vi "Merge Image Data with mask.vi"(6 "Col":i32=1, 7 "Row":i32=1, 9 "Mask":u8[][](array[numeric])=[[0, 1, 1], [1, 0, 1], [1, 1, 1]], 10 "Image Data 2":u16[][](array[numeric])=[[2, 2, 2], [2, 2, 2], [2, 2, 2]] format="%.0x", 11 "Image Data 1":u16[][](array[numeric])=[[0, 0, 0, 0, 0, 0, 0, 0, 0, 0, 0, 0, 0, 0, 0, 0], [0, 3, 3, 3, 0, 0, 0, 0, 0, 0, 0, 0, 0, 0, 0, 0], [0, 3, 3, 3, 0, 0, 0, 0, 0, 0, 0, 0, 0, 0, 0, 0], [0, 3, 3, 3, 0, 0, 0, 0, 0, 0, 0, 0, 0, 0, 0, 0], [0, 0, 0, 0, 0, 0, 0, 0, 0, 0, 0, 0, 0, 0, 0, 0], [0, 0, 0, 0, 0, 0, 0, 0, 0, 0, 0, 0, 0, 0, 0, 0], [0, 0, 0, 0, 0, 0, 0, 0, 0, 0, 0, 0, 0, 0, 0, 0], [0, 0, 0, 0, 0, 0, 0, 0, 0, 0, 0, 0, 0, 0, 0, 0], [0, 0, 0, 0, 0, 0, 0, 0, 0, 0, 0, 0, 0, 0, 0, 0]] format="%.0x") -> (3 "Merged Data":u16[][](array[numeric]) format="%.0x")   [LabVIEW 2019]
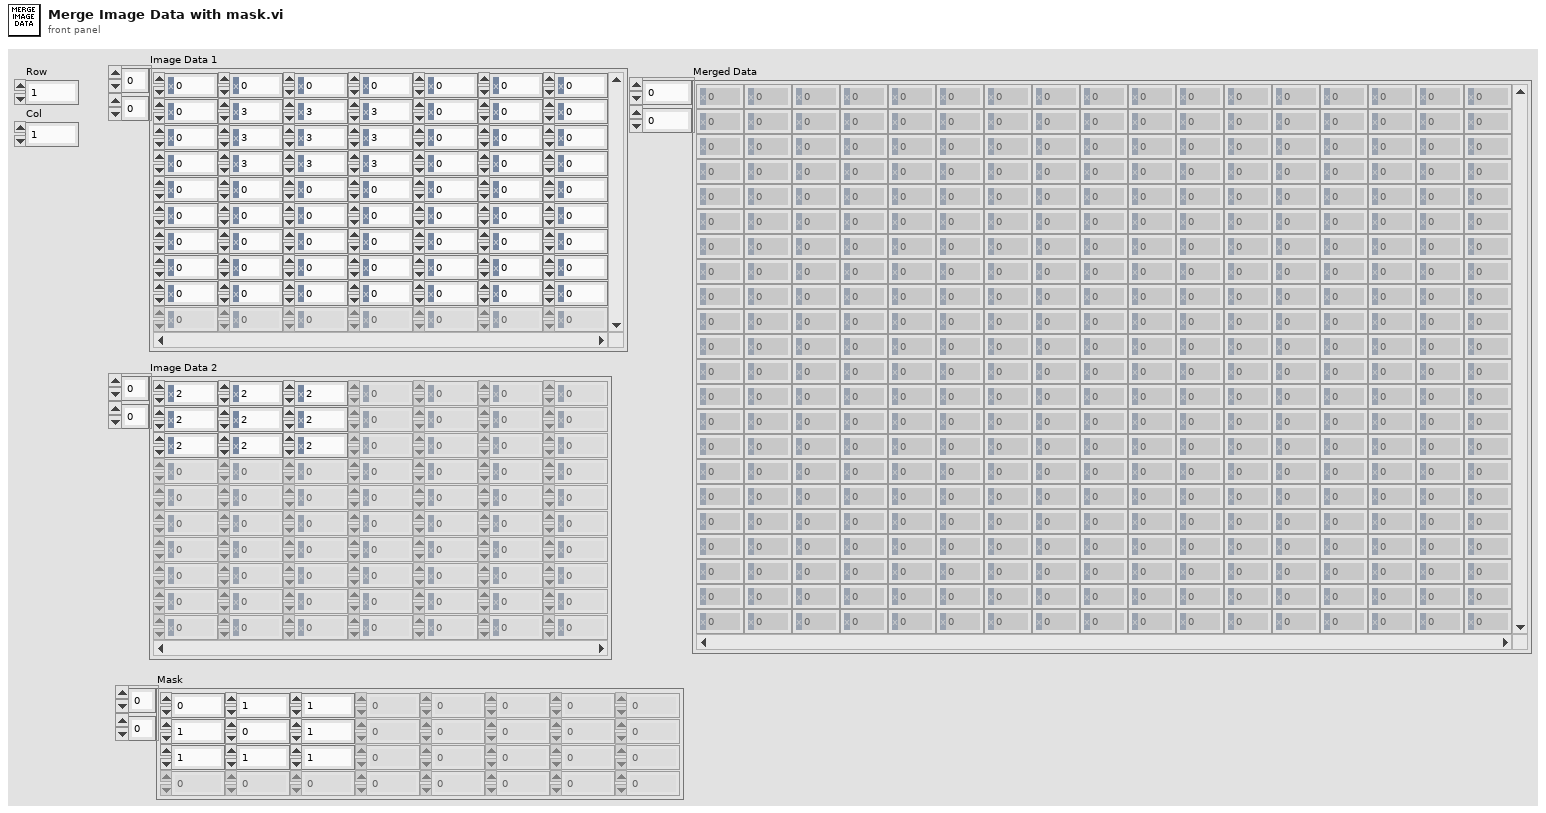
[diagram p1: front panel]
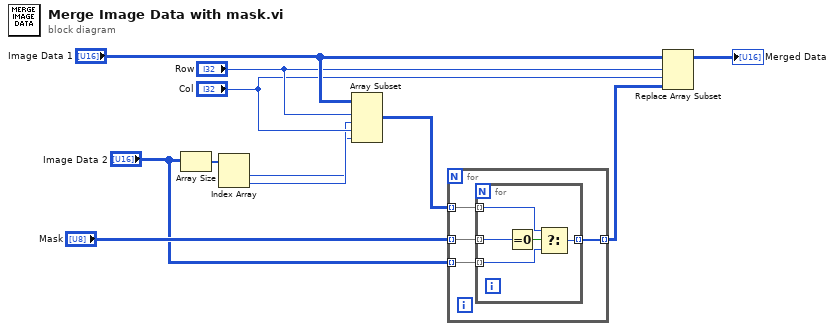
[diagram p0: block diagram]
diagram:
  n1 = Array Size(array="Image Data 2") -> (size(s)=w8:i32[])
  n2 = Index Array(array=w8) -> (element #1=w1:i32, element #2=w2:i32)  [unwired: 2 in]
  n3 = Array Subset(array="Image Data 1", index (row)="Row", length (row)=w2, index (col)="Col", length (col)=w1) -> (w7:u16[][])
  n4 = for {
    tunnel: w7 -> [w15] mode=indexing
    tunnel: "Mask" -> [w14] mode=indexing
    tunnel: "Image Data 2" -> [w13] mode=indexing
    tunnel: [w12] -> w4 mode=indexing
    n5 = for {
      tunnel: w15 -> [w18] mode=indexing
      tunnel: w14 -> [w19] mode=indexing
      tunnel: w13 -> [w17] mode=indexing
      tunnel: [w16] -> w12 mode=indexing
      n6 = Equal To 0?(x=w19) -> (x = 0?=w20:bool)
      n7 = Select(t=w18, s=w20, f=w17) -> (s? t:f=w16:u16)
    }
  }
  n8 = Replace Array Subset(array="Image Data 1", new element=w4, index (row)="Row", index (col)="Col") -> (→"Merged Data":u16[][])
